vi "Switch Directions.vi"(11 "input cluster":T1) -> (2 "Yout":dbl, 3 "Xout":dbl)   [LabVIEW 2016]
uses:
  Controls.ctl
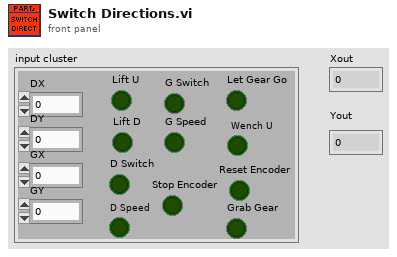
[diagram p1: front panel]
types:
  T1 = typedef "Controls.ctl" = cluster{"DX":dbl, "DY":dbl, "GX":dbl, "GY":dbl, "Lift U":bool, "D Switch":bool, "D Speed":bool, "G Switch":bool, "G Speed":bool, " Wench U":bool, "Lift D":bool, "Let Gear Go":bool, "Grab Gear":bool, "Reset Encoder":bool, "Stop Encoder":bool}
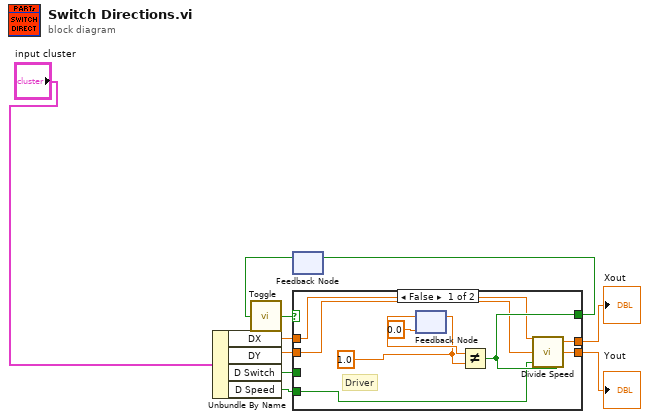
[diagram p0: block diagram]
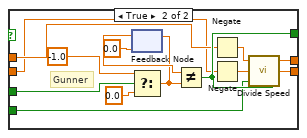
[diagram p2: hidden frame]
diagram:
  n1 = Unbundle By Name("input cluster") -> ("DX"=w8:dbl, "DY"=w9:dbl, "D Switch"=w6:bool, "D Speed"=w7:bool)
  n2 = feedback #1() -> (w3:bool)  [unwired: 1 in]
  n3 = call "Toggle.vi"("Input"=w3) -> ("Output"=w2:bool)  [unwired: 4 in]
  n4 = case shown="False" w2 {
    tunnel: [w15 w26] -> w1
    tunnel: [w17 w28] -> w4
    tunnel: [w16 w27] -> w5
    tunnel: w6 -> [_ w23]
    tunnel: w7 -> [w14 w22]
    tunnel: w8 -> [w13 w21]
    tunnel: w9 -> [w12 w20]
    frame False {
      w11 = 1.0 ("t")
      # "Driver"
      n5 = feedback #2(0.0 ("t")) -> (w19:dbl)
      n6 = feedback-in #2(w11) -> ()
      n7 = Not Equal?(x=w19, y=w11) -> (x != y?=w15:bool)
      n8 = call "Divide Speed.vi"("Reset"=w15, "Speed"=w14, "Y"=w12, "X"=w13) -> ("Yout"=w16:dbl, "Xout"=w17:dbl)
    }
    frame True {
      # "Gunner"
      n9 = feedback #3(0.0 ("t")) -> (w30:dbl)
      n10 = Select(t=-1.0, s=w23, f=0.0) -> (s? t:f=w29:dbl)
      n11 = feedback-in #3(w29) -> ()
      n12 = Not Equal?(x=w30, y=w29) -> (x != y?=w26:bool)
      n13 = Negate(x=w21) -> (-x=w25:dbl)
      n14 = Negate(x=w20) -> (-x=w24:dbl)
      n15 = call "Divide Speed.vi"("Reset"=w26, "Speed"=w22, "Y"=w24, "X"=w25) -> ("Yout"=w27:dbl, "Xout"=w28:dbl)
    }
  }
  "Yout" <- w5
  "Xout" <- w4
  n16 = feedback-in #1(w1) -> ()
